vi "SENS_CORR_COLL_GUID_CKIT_PORT.vi"(0 "VISA IN":refnum<visa-resource-name>, 5 "error in":errorcluster, 6 "Ecal ID":string="APC 3.5 female", 7 "Channel":i32, 9 "Port":i32=1) -> (14 "VISA Out":refnum<visa-resource-name>, 19 "error out":errorcluster)   [LabVIEW 2018, in "PNA-X.lvlib"]
doc: "SENSe:CORRection:COLLect:GUIDed:CKIT:PORT<pnum>[:SELect] <kit> \n(Read-Write) Specifies the calibration kit for each port to be used during a guided calibration. An unused port does NOT need to have a specified Cal Kit. \n\nIf two or more identical ECal modules are connected to the PNA, the serial number must be included in the <kit> string to distinguish the ECal modules. See SENS:CORR:COLL:GUID:CKIT:PORT:CAT?\n\nNote: Sliding loads are not fully supported from Sens:Corr:Coll:Guided... The Measure button must be manually pressed.\n\n \n\n1. Specify the connector type for the port with SENS:CORR:COLL:GUID:CONN:PORT. \n\n2. Query the valid available kits for the connector on each port with SENS:CORR:COLL:GUID:CKIT:PORT:CAT?\n\n3. Specify the kit using this command.\n\n4. Perform a query of this command. If the <kit> parameter was incorrectly entered, an error will be returned.\n \nParameters\n \n \n<pnum>\n Any existing port number. If unspecified, value is set to 1\n \n<kit>\n Calibration kit to be used for the specified port.\n \nExamples\n SENS:CORR:COLL:GUID:CKIT:PORT1 '85055A'\n'The following includes a serial number when two or more ECal mods are connected\nsense:correction:collect:guided:ckit:port2:select '85092-60010 ECal 10685'\n \nQuery Syntax\n SENSe:CORRection:COLLect:GUIDed:CKIT:PORT<pnum>[:SELect]?\n \nReturn Type\n String - If the <kit> parameter was incorrectly entered while writing, an error will be returned.\n \nDefault\n Not Applicable"
uses:
  PNA-X.lvlib
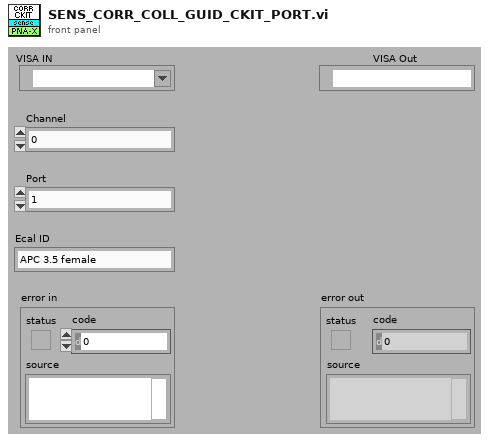
[diagram p1: front panel]
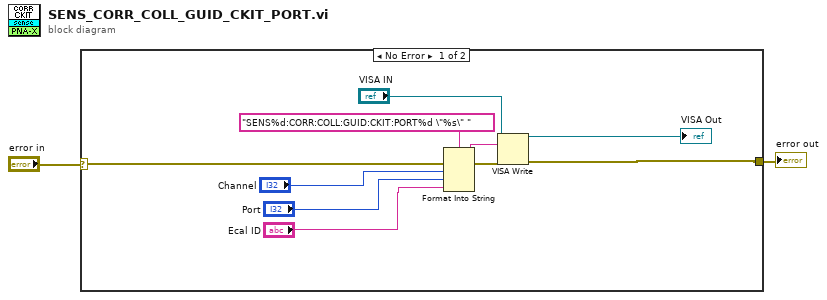
[diagram p0: block diagram]
diagram:
  n1 = case shown="No Error" "error in" {
    selector: "error in" -> [w12 w13]
    tunnel: [w7 w13] -> w1
    frame No Error {
      n2 = Format Into String(format string="SENS%d:CORR:COLL:GUID:CKIT:PORT%d \"%s\" " ("Cmdline"), error in=w12, "Channel", "Port", "Ecal ID") -> (resulting string=w10:string, error out=w11:errorcluster)  [unwired: 1 in]
      n3 = VISA Write(VISA resource name="VISA IN", write buffer=w10, error in (no error)=w11) -> (VISA resource name out=→"VISA Out":refnum<visa-resource-name>, error out=w7:errorcluster)  [unwired: 1 out]
    }
    frame Error {
    }
  }
  "error out" <- w1
